vi "Monitor-filters.vi"(8 "error in":errorcluster, 9 "Temperature characteristics":T1 {"Stand. dev. temperature" format="%#.1f"; "Min. temperature" format="%#.0f"; "Max. temperature" format="%#.0f"; "Average temperature" format="%#.0f"}, 10 "Characteristics":T2[](array[typedef]), 11 "Filter params. ref. in":refnum<data-value>) -> (0 "error IO":errorcluster, 1 "Add to report?":bool, 3 "Filter params. ref.":refnum<data-value>)   [LabVIEW 2013, in "CameraVision.lvlib" / "CV-Filter.lvclass"]
uses:
  CV-Filter.lvclass
  Analysis/Characteristics-cluster.ctl
  Temperature/Temperature-characteristics.ctl
  CV-Filter.lvclass/CV-Filter.ctl
  Read Filter array temp.vi
  Read Duration temp.vi
  Write Duration temp.vi
  Write Values temp.vi
  Analysis/CV-Analysis.lvclass
  Temperature/CV-Temperature.lvclass
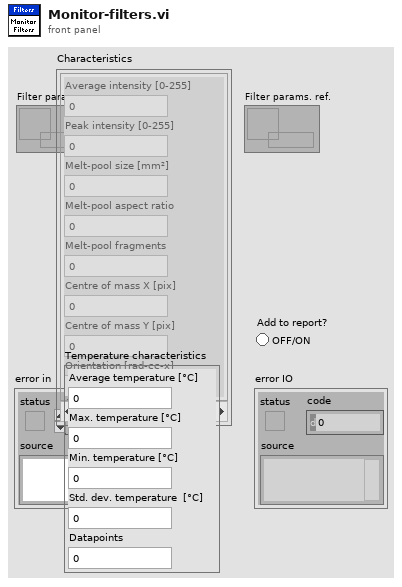
[diagram p1: front panel]
types:
  T1 = typedef "CameraVision.lvlib/CV-Temperature.lvclass/Temperature-characteristics.ctl" = cluster{"Average temperature ":dbl, "Max. temperature":dbl, "Min. temperature":dbl, "Stand. dev. temperature":dbl, "Datapoints":dbl}
  T2 = typedef "CameraVision.lvlib/CV-Analysis.lvclass/Characteristics-cluster.ctl" = cluster{"Average intensity":dbl, "Peak intensity":dbl, "Melt-pool size":dbl, "Melt-pool aspect ratio":dbl, "Melt-pool fragments":dbl, "Centre of mass X":dbl, "Centre of mass Y":dbl, "Orientation":dbl}
  T3 = typedef "Filter.ctl" = cluster{"Characteristic":T4, "Monitor":bool, "Min.":dbl, "Max.":dbl, "Min. Thres.":dbl, "Min. Dur.":u16, "Report":bool}
  T4 = typedef "Filter-characteristic.ctl" = enum16{"Average intensity [0-255]", "Peak intensity [0-255]", "Melt-pool size [mm²]", "Melt-pool aspect ratio []", "Melt-pool fragments []", "Melt-pool position X [pixel]", "Melt-pool position Y [pixel]", "Average temperature [°C]", "Max. temperature [°C]", "Min. temperature [°C]", "Std. dev. temperature [°C]"}
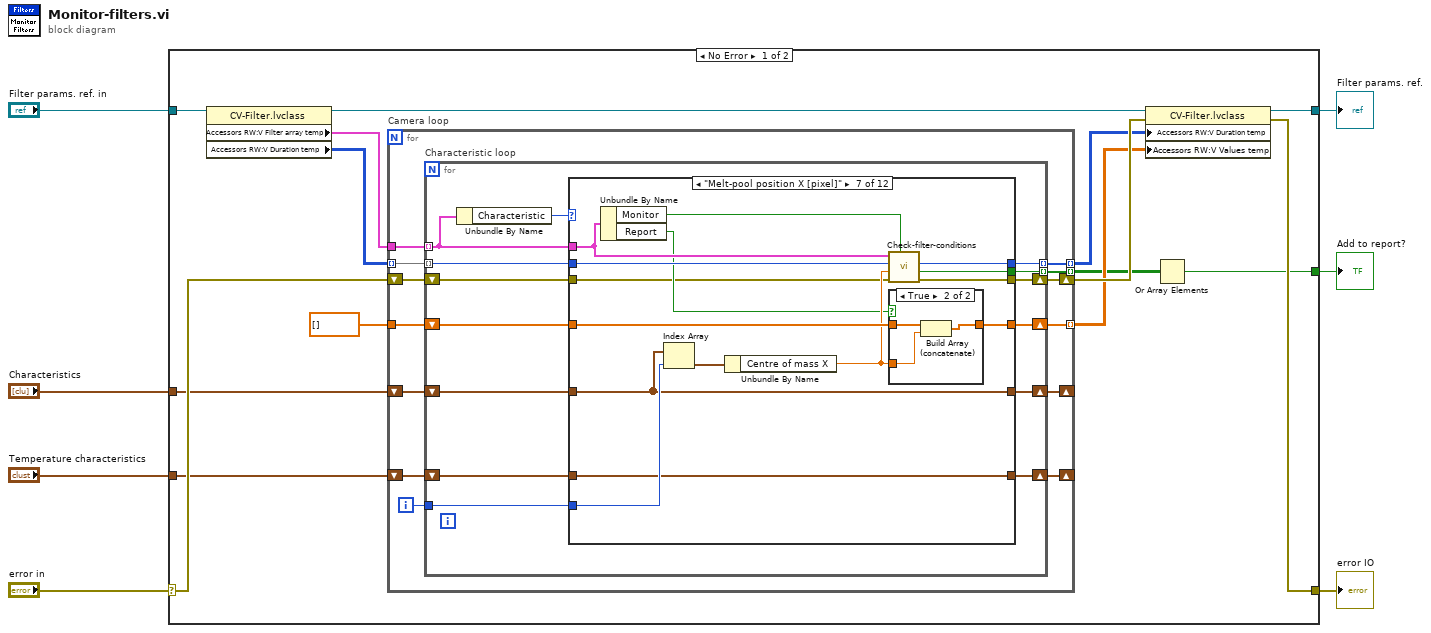
[diagram p0: block diagram]
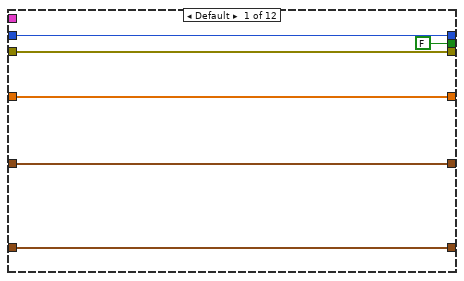
[diagram p2: hidden frame]
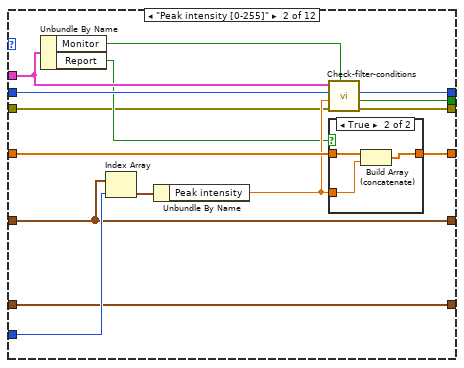
[diagram p3: hidden frame]
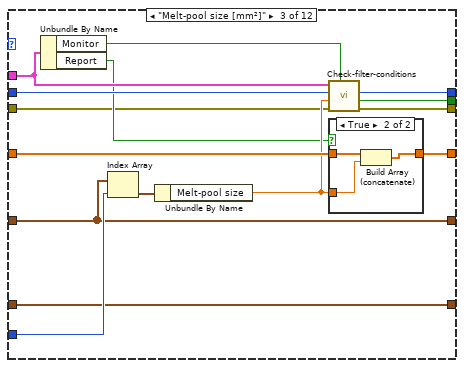
[diagram p5: hidden frame]
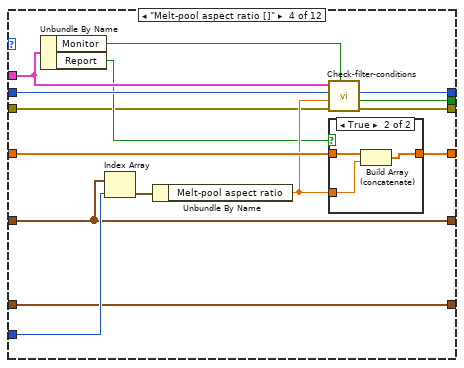
[diagram p7: hidden frame]
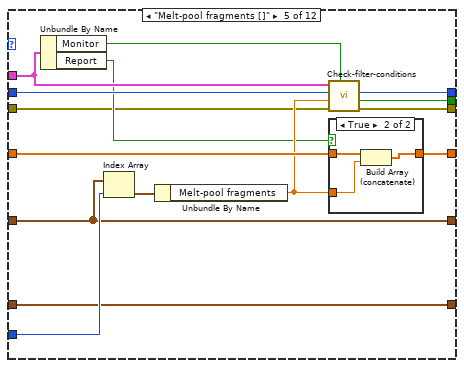
[diagram p9: hidden frame]
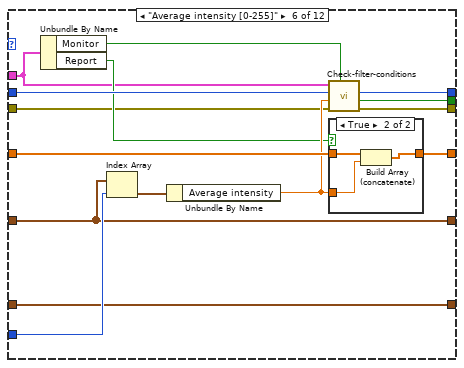
[diagram p11: hidden frame]
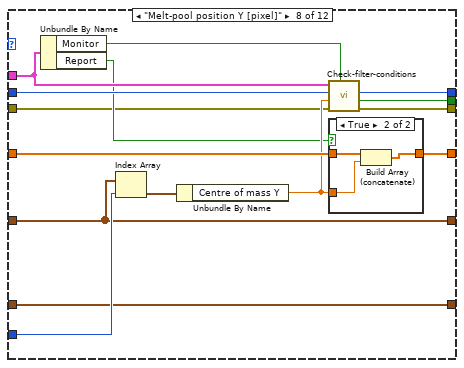
[diagram p14: hidden frame]
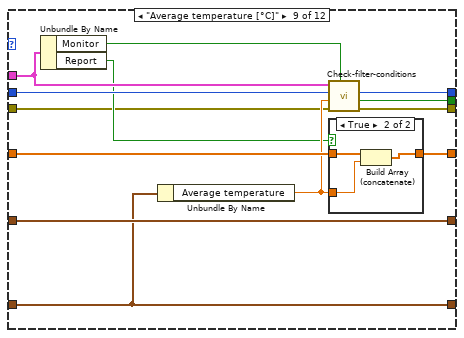
[diagram p16: hidden frame]
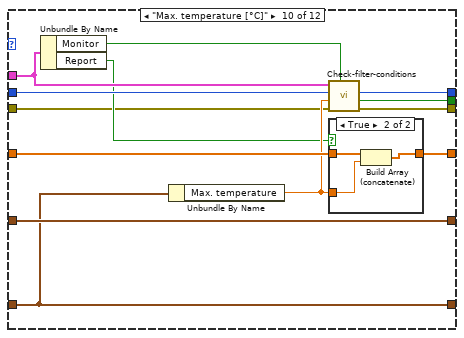
[diagram p18: hidden frame]
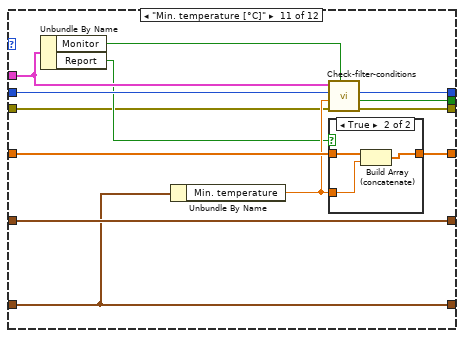
[diagram p20: hidden frame]
diagram:
  n1 = case shown="No Error" "error in" {
    selector: "error in" -> [w10 w258]
    tunnel: "Filter params. ref. in" -> [w21 w259]
    tunnel: [w14 w259] -> w6
    tunnel: [w13 w258] -> w5
    tunnel: [w11 FALSE ("Boolean")] -> w4
    tunnel: "Temperature characteristics" -> [w9 _]
    tunnel: "Characteristics" -> [w8 _]
    frame No Error {
      n2 = property class="CV-Filter.lvclass"(reference=w21) -> (reference out=w18:refnum<data-value>, "Accessors RW:V Filter array temp"=w20:T3[], "Accessors RW:V Duration temp"=w19:u16[][])  [unwired: 1 in, 1 out]
      n3 = for "Camera loop" {
        tunnel: w20 -> [w35]
        tunnel: w19 -> [w34] mode=indexing
        shift-right: [w29] -> _
        shift-left: w8 -> [w32]
        shift-right: [w28] -> _
        shift-left: w9 -> [w33]
        tunnel: [w27] -> w16 mode=indexing
        tunnel: dbl[] [] -> [w26]
        tunnel: [w25] -> w12 mode=indexing
        shift-right: [w24] -> w17
        shift-left: w10 -> [w31]
        tunnel: [w23] -> w15 mode=indexing
        i -> [w30]
        n4 = for "Characteristic loop" {
          tunnel: w35 -> [w48] mode=indexing
          tunnel: w34 -> [w47] mode=indexing
          shift-right: [w43] -> w29
          shift-left: w32 -> [w46]
          shift-right: [w36] -> w28
          shift-left: w33 -> [w37]
          tunnel: w30 -> [w44]
          tunnel: [w42] -> w27 mode=indexing
          shift-right: [w40] -> w23
          shift-left: w26 -> [w41]
          tunnel: [w39] -> w25 mode=indexing
          shift-right: [w38] -> w24
          shift-left: w31 -> [w45]
          n5 = Unbundle By Name(w48) -> ("Characteristic"=w49:T4)
          n6 = case shown="\"Melt-pool position X [pixel]\"" w49 {
            tunnel: w48 -> [_ w66 w85 w104 w123 w134 w161 w180 w199 w216 w233 w250]
            tunnel: w47 -> [w55 w64 w83 w102 w121 w141 w159 w178 w197 w214 w231 w248]
            tunnel: w46 -> [w51 w57 w76 w95 w114 w133 w152 w171 w191 w208 w225 w242]
            tunnel: w45 -> [w54 w56 w75 w94 w113 w132 w151 w170 w190 w207 w224 w241]
            tunnel: w44 -> [_ w70 w89 w108 w127 w146 w165 w184 _ _ _ _]
            tunnel: [w54 w68 w87 w106 w125 w144 w163 w182 w201 w218 w235 w252] -> w38
            tunnel: [w55 w67 w86 w105 w124 w143 w162 w181 w200 w217 w234 w251] -> w42
            tunnel: [w51 w57 w76 w95 w114 w133 w152 w171 w191 w208 w225 w242] -> w43
            tunnel: [FALSE ("Alert?") w63 w82 w101 w120 w140 w158 w177 w196 w213 w230 w247] -> w39
            tunnel: w41 -> [w53 w62 w81 w100 w119 w139 w157 w176 w195 w212 w229 w246]
            tunnel: [w53 w60 w79 w98 w117 w137 w155 w174 w193 w210 w227 w244] -> w40
            tunnel: w37 -> [w50 w58 w77 w96 w115 w135 w153 w172 w189 w206 w223 w240]
            tunnel: [w50 w58 w77 w96 w115 w135 w153 w172 w189 w206 w223 w240] -> w36
            frame Default {
            }
            frame "Peak intensity [0-255]" {
              n7 = Unbundle By Name(w66) -> ("Monitor"=w65:bool, "Report"=w59:bool)
              n8 = Index Array(array=w57, index=w70) -> (element=w69:T2)
              n9 = Unbundle By Name(w69) -> ("Peak intensity"=w61:dbl)
              n10 = call "Check-filter-conditions.vi"("Monitor"=w65, "error in"=w56, "Value"=w61, "Duration in"=w64, "Conditions"=w66) -> ("error"=w68:errorcluster, "Alert?"=w63:bool, "Duration"=w67:u16)  [unwired: 4 in]
              n11 = case shown="True" w59 {
                tunnel: w62 -> [w71 w74]
                tunnel: w61 -> [_ w73]
                tunnel: [w71 w72] -> w60
                frame False {
                }
                frame True {
                  n12 = Build Array (concatenate)(w74, w73) -> (w72:dbl[])
                }
              }
            }
            frame "Melt-pool size [mm²]" {
              n13 = Unbundle By Name(w85) -> ("Monitor"=w84:bool, "Report"=w78:bool)
              n14 = Index Array(array=w76, index=w89) -> (element=w88:T2)
              n15 = Unbundle By Name(w88) -> ("Melt-pool size"=w80:dbl)
              n16 = call "Check-filter-conditions.vi"("Monitor"=w84, "error in"=w75, "Value"=w80, "Duration in"=w83, "Conditions"=w85) -> ("error"=w87:errorcluster, "Alert?"=w82:bool, "Duration"=w86:u16)  [unwired: 4 in]
              n17 = case shown="True" w78 {
                tunnel: w81 -> [w90 w93]
                tunnel: w80 -> [_ w92]
                tunnel: [w90 w91] -> w79
                frame False {
                }
                frame True {
                  n18 = Build Array (concatenate)(w93, w92) -> (w91:dbl[])
                }
              }
            }
            frame "Melt-pool aspect ratio []" {
              n19 = Unbundle By Name(w104) -> ("Monitor"=w103:bool, "Report"=w97:bool)
              n20 = Index Array(array=w95, index=w108) -> (element=w107:T2)
              n21 = Unbundle By Name(w107) -> ("Melt-pool aspect ratio"=w99:dbl)
              n22 = call "Check-filter-conditions.vi"("Monitor"=w103, "error in"=w94, "Value"=w99, "Duration in"=w102, "Conditions"=w104) -> ("error"=w106:errorcluster, "Alert?"=w101:bool, "Duration"=w105:u16)  [unwired: 4 in]
              n23 = case shown="True" w97 {
                tunnel: w100 -> [w109 w112]
                tunnel: w99 -> [_ w111]
                tunnel: [w109 w110] -> w98
                frame False {
                }
                frame True {
                  n24 = Build Array (concatenate)(w112, w111) -> (w110:dbl[])
                }
              }
            }
            frame "Melt-pool fragments []" {
              n25 = Unbundle By Name(w123) -> ("Monitor"=w122:bool, "Report"=w116:bool)
              n26 = Index Array(array=w114, index=w127) -> (element=w126:T2)
              n27 = Unbundle By Name(w126) -> ("Melt-pool fragments"=w118:dbl)
              n28 = call "Check-filter-conditions.vi"("Monitor"=w122, "error in"=w113, "Value"=w118, "Duration in"=w121, "Conditions"=w123) -> ("error"=w125:errorcluster, "Alert?"=w120:bool, "Duration"=w124:u16)  [unwired: 4 in]
              n29 = case shown="True" w116 {
                tunnel: w119 -> [w128 w131]
                tunnel: w118 -> [_ w130]
                tunnel: [w128 w129] -> w117
                frame False {
                }
                frame True {
                  n30 = Build Array (concatenate)(w131, w130) -> (w129:dbl[])
                }
              }
            }
            frame "Average intensity [0-255]" {
              n31 = Unbundle By Name(w134) -> ("Monitor"=w142:bool, "Report"=w136:bool)
              n32 = Index Array(array=w133, index=w146) -> (element=w145:T2)
              n33 = Unbundle By Name(w145) -> ("Average intensity"=w138:dbl)
              n34 = call "Check-filter-conditions.vi"("Monitor"=w142, "error in"=w132, "Value"=w138, "Duration in"=w141, "Conditions"=w134) -> ("error"=w144:errorcluster, "Alert?"=w140:bool, "Duration"=w143:u16)  [unwired: 4 in]
              n35 = case shown="True" w136 {
                tunnel: w139 -> [w147 w150]
                tunnel: w138 -> [_ w149]
                tunnel: [w147 w148] -> w137
                frame False {
                }
                frame True {
                  n36 = Build Array (concatenate)(w150, w149) -> (w148:dbl[])
                }
              }
            }
            frame "Melt-pool position X [pixel]" {
              n37 = Unbundle By Name(w161) -> ("Monitor"=w160:bool, "Report"=w154:bool)
              n38 = Index Array(array=w152, index=w165) -> (element=w164:T2)
              n39 = Unbundle By Name(w164) -> ("Centre of mass X"=w156:dbl)
              n40 = call "Check-filter-conditions.vi"("Monitor"=w160, "error in"=w151, "Value"=w156, "Duration in"=w159, "Conditions"=w161) -> ("error"=w163:errorcluster, "Alert?"=w158:bool, "Duration"=w162:u16)  [unwired: 4 in]
              n41 = case shown="True" w154 {
                tunnel: w157 -> [w166 w169]
                tunnel: w156 -> [_ w168]
                tunnel: [w166 w167] -> w155
                frame False {
                }
                frame True {
                  n42 = Build Array (concatenate)(w169, w168) -> (w167:dbl[])
                }
              }
            }
            frame "Melt-pool position Y [pixel]" {
              n43 = Unbundle By Name(w180) -> ("Monitor"=w179:bool, "Report"=w173:bool)
              n44 = Index Array(array=w171, index=w184) -> (element=w183:T2)
              n45 = Unbundle By Name(w183) -> ("Centre of mass Y"=w175:dbl)
              n46 = call "Check-filter-conditions.vi"("Monitor"=w179, "error in"=w170, "Value"=w175, "Duration in"=w178, "Conditions"=w180) -> ("error"=w182:errorcluster, "Alert?"=w177:bool, "Duration"=w181:u16)  [unwired: 4 in]
              n47 = case shown="True" w173 {
                tunnel: w176 -> [w185 w188]
                tunnel: w175 -> [_ w187]
                tunnel: [w185 w186] -> w174
                frame False {
                }
                frame True {
                  n48 = Build Array (concatenate)(w188, w187) -> (w186:dbl[])
                }
              }
            }
            frame "Average temperature [°C]" {
              n49 = Unbundle By Name(w199) -> ("Monitor"=w198:bool, "Report"=w192:bool)
              n50 = Unbundle By Name(w189) -> ("Average temperature"=w194:dbl)
              n51 = call "Check-filter-conditions.vi"("Monitor"=w198, "error in"=w190, "Value"=w194, "Duration in"=w197, "Conditions"=w199) -> ("error"=w201:errorcluster, "Alert?"=w196:bool, "Duration"=w200:u16)  [unwired: 4 in]
              n52 = case shown="True" w192 {
                tunnel: w195 -> [w202 w205]
                tunnel: w194 -> [_ w204]
                tunnel: [w202 w203] -> w193
                frame False {
                }
                frame True {
                  n53 = Build Array (concatenate)(w205, w204) -> (w203:dbl[])
                }
              }
            }
            frame "Max. temperature [°C]" {
              n54 = Unbundle By Name(w216) -> ("Monitor"=w215:bool, "Report"=w209:bool)
              n55 = Unbundle By Name(w206) -> ("Max. temperature"=w211:dbl)
              n56 = call "Check-filter-conditions.vi"("Monitor"=w215, "error in"=w207, "Value"=w211, "Duration in"=w214, "Conditions"=w216) -> ("error"=w218:errorcluster, "Alert?"=w213:bool, "Duration"=w217:u16)  [unwired: 4 in]
              n57 = case shown="True" w209 {
                tunnel: w212 -> [w219 w222]
                tunnel: w211 -> [_ w221]
                tunnel: [w219 w220] -> w210
                frame False {
                }
                frame True {
                  n58 = Build Array (concatenate)(w222, w221) -> (w220:dbl[])
                }
              }
            }
            frame "Min. temperature [°C]" {
              n59 = Unbundle By Name(w233) -> ("Monitor"=w232:bool, "Report"=w226:bool)
              n60 = Unbundle By Name(w223) -> ("Min. temperature"=w228:dbl)
              n61 = call "Check-filter-conditions.vi"("Monitor"=w232, "error in"=w224, "Value"=w228, "Duration in"=w231, "Conditions"=w233) -> ("error"=w235:errorcluster, "Alert?"=w230:bool, "Duration"=w234:u16)  [unwired: 4 in]
              n62 = case shown="True" w226 {
                tunnel: w229 -> [w236 w239]
                tunnel: w228 -> [_ w238]
                tunnel: [w236 w237] -> w227
                frame False {
                }
                frame True {
                  n63 = Build Array (concatenate)(w239, w238) -> (w237:dbl[])
                }
              }
            }
            frame "Std. dev. temperature [°C]" {
              n64 = Unbundle By Name(w250) -> ("Monitor"=w249:bool, "Report"=w243:bool)
              n65 = Unbundle By Name(w240) -> ("Stand. dev. temperature"=w245:dbl)
              n66 = call "Check-filter-conditions.vi"("Monitor"=w249, "error in"=w241, "Value"=w245, "Duration in"=w248, "Conditions"=w250) -> ("error"=w252:errorcluster, "Alert?"=w247:bool, "Duration"=w251:u16)  [unwired: 4 in]
              n67 = case shown="True" w243 {
                tunnel: w246 -> [w253 w256]
                tunnel: w245 -> [_ w255]
                tunnel: [w253 w254] -> w244
                frame False {
                }
                frame True {
                  n68 = Build Array (concatenate)(w256, w255) -> (w254:dbl[])
                }
              }
            }
          }
        }
      }
      n69 = property class="CV-Filter.lvclass"(reference=w18, error in=w17, "Accessors RW:V Duration temp"=w16, "Accessors RW:V Values temp"=w15) -> (reference out=w14:refnum<data-value>, error out=w13:errorcluster)
      n70 = Or Array Elements(Boolean array=w12) -> (logical OR=w11:bool)
    }
    frame Error {
    }
  }
  "Filter params. ref." <- w6
  "error IO" <- w5
  "Add to report?" <- w4
